vi "tm_preparecapture_40.vi"(8 "error in (no error)":errorcluster {"code" format="%.0x"}, 9 "Frames":i32, 10 "Capture mode":i32(ring) items=["Snap", "Sequence"], 11 "Handle in":u32) -> (0 "error out":errorcluster {"code" format="%.0x"}, 2 "Buffer Info":T1, 3 "Handle out":u32, 4 "Image type":u32)   [LabVIEW 2023]
uses:
  tmcamcon.dll
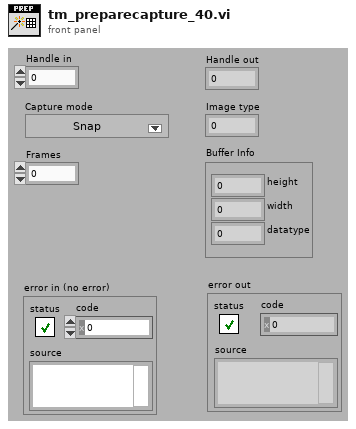
[diagram p1: front panel]
types:
  T1 = cluster{"height":i32, "width":i32, "datatype":i32}
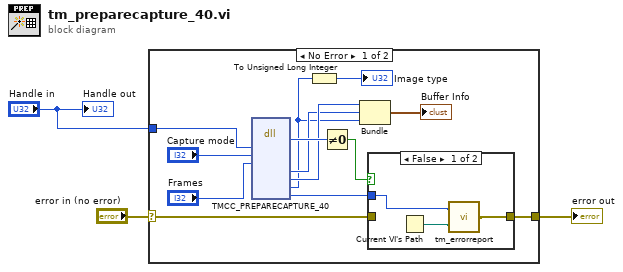
[diagram p0: block diagram]
diagram:
  n1 = case shown="No Error" "error in (no error)" {
    selector: "error in (no error)" -> [w9 w21]
    tunnel: [w6 w21] -> w1
    tunnel: "Handle in" -> [w15 _]
    frame No Error {
      n2 = dll-call lib="tmcamcon.dll" fn="TMCC_PREPARECAPTURE_40"("index"=w15, "mode"="Capture mode", "frames"="Frames") -> ("return type"=w16:u32, "width"=w11:i32, "height"=w12:i32, "datatype"=w4:i32, "Erval"=w8:i32)  [unwired: 10 in, 2 out]
      n3 = To Unsigned Long Integer(number=w4) -> (unsigned 32bit integer=→"Image type":u32)
      n4 = Not Equal To 0?(x=w16) -> (x != 0?=w7:bool)
      n5 = Bundle("height"=w12, "width"=w11, "datatype"=w4) -> (→"Buffer Info":T1)  [unwired: 1 in]
      n6 = case shown="False" w7 {
        tunnel: w9 -> [_ w20]
        tunnel: [w17 w20] -> w6
        tunnel: w8 -> [w18 _]
        frame False {
          n7 = Current VI's Path() -> (path=w19:path)
          n8 = call "tm_errorreport.vi"("Source"=w19, "Error"=w18) -> ("error out"=w17:errorcluster)
        }
        frame True {
        }
      }
    }
    frame Error {
    }
  }
  "error out" <- w1
  "Handle out" <- "Handle in"
